vi "AlliGator Compute (1-G2_INT)xMean(INT) Images.vi"(4 "INT Images":T1[](array[typedef]), 6 "Sum(INT)":T1, 7 "G2 Images":T1[](array[typedef]), 8 "Error In":errorcluster, 9 "Min(G2)":T1, 10 "Max(G2)":T1, 11 "Sum(G2)":T1) -> (0 "Error Out":errorcluster, 1 "Min((1-G2/INT)*<INT>)":T1, 2 "Max((1-G2/INT)*<INT>)":T1, 3 "Sum((1-G2/INT)*<INT>)":T1, 5 "(1-G2/INT)*<INT> Images":T1[](array[typedef]))   [LabVIEW 2021, in "AlliGator Dual-Channel Datasets.lvlib"]
doc: "Computes (1 - G2/INT)*<INT>."
uses:
  AlliGator Dual-Channel Datasets.lvlib
  <vilib>/vision/Image Controls.llb/IMAQ Image.ctl
  <vilib>/vision/NI_Vision_Development_Module.lvlib
  Image/Image.lvlib
  Utilities/Utilities.lvlib
panel:
  # "see the AlliGator License on the block diagram (Ctrl+E or Window:Show Block Diagram)"
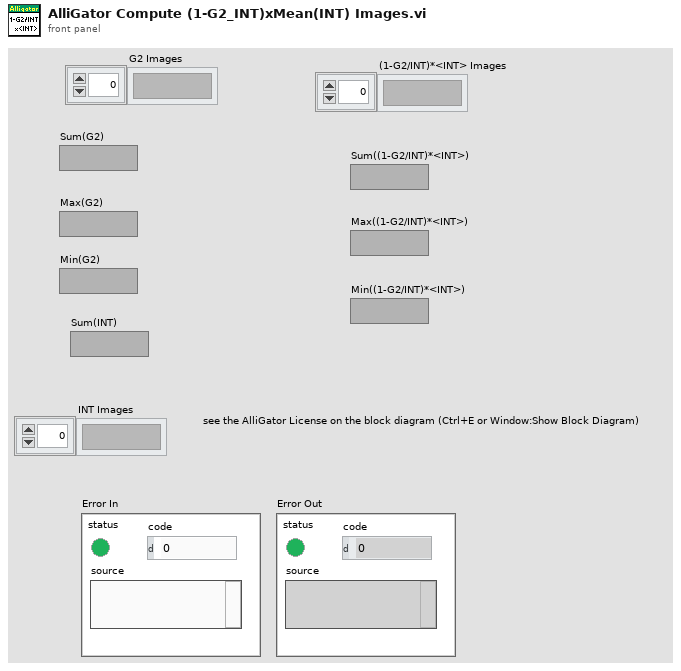
[diagram p1: front panel]
types:
  T1 = typedef "IMAQ Image.ctl" = refnum<image>
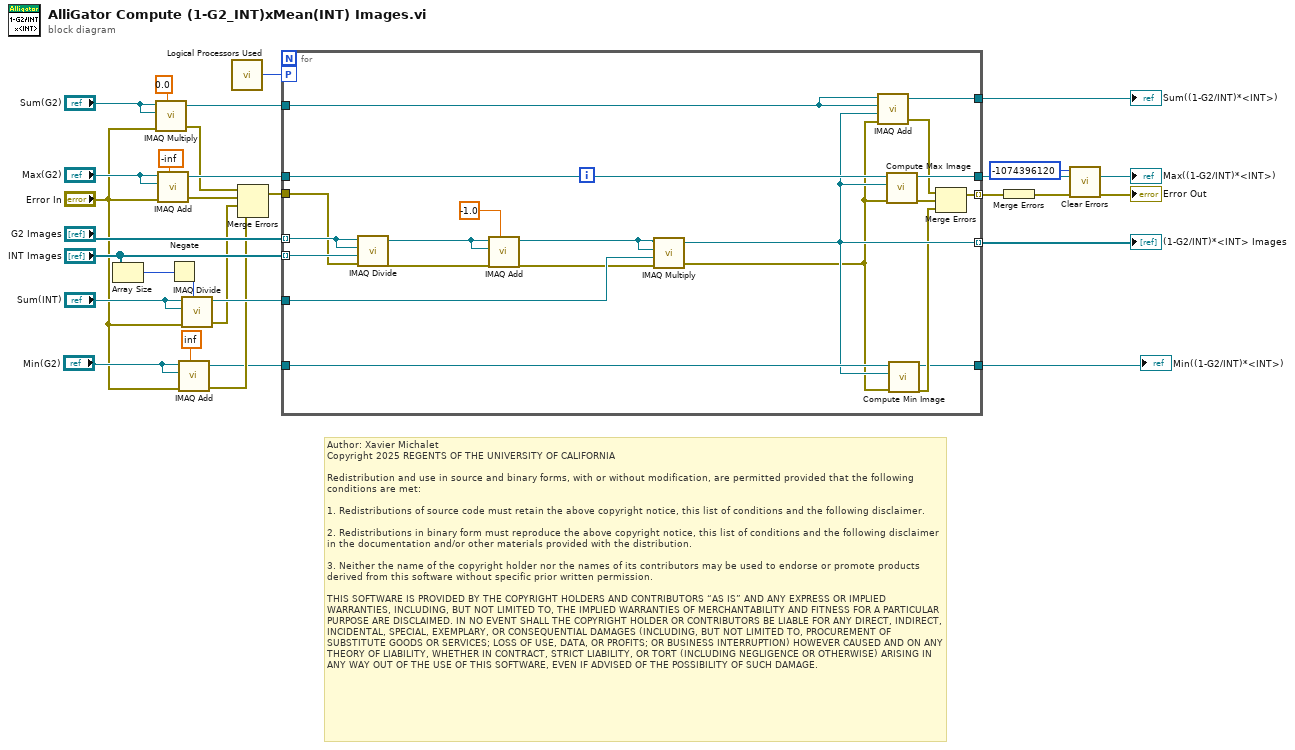
[diagram p0: block diagram]
diagram:
  # "Author: Xavier Michalet\nCopyright 2025 REGENTS OF THE UNIVERSITY OF CALIFORNIA\n\nRedistribution and use in source and binary forms, with or without modification, are permitted provided that the following conditions are met:\n\n1. Redistributions of source code must retain the above copyright notice, this list of conditions and the following disclaimer.\n\n2. Redistributions in binary form must reproduce the above copyright notice, this list of conditions and the following disclaimer in the documentation and/or other materials provided with the distribution.\n\n3. Neither the name of the copyright holder nor the names of its contributors may be used to endorse or promote products derived from this software without specific prior written permission.\n\nTHIS SOFTWARE IS PROVIDED BY THE COPYRIGHT HOLDERS AND CONTRIBUTORS “AS IS” AND ANY EXPRESS OR IMPLIED WARRANTIES, INCLUDING, BUT NOT LIMITED TO, THE IMPLIED WARRANTIES OF MERCHANTABILITY AND FITNESS FOR A PARTICULAR PURPOSE ARE DISCLAIMED. IN NO EVENT SHALL THE COPYRIGHT HOLDER OR CONTRIBUTORS BE LIABLE FOR ANY DIRECT, INDIRECT, INCIDENTAL, SPECIAL, EXEMPLARY, OR CONSEQUENTIAL DAMAGES (INCLUDING, BUT NOT LIMITED TO, PROCUREMENT OF SUBSTITUTE GOODS OR SERVICES; LOSS OF USE, DATA, OR PROFITS; OR BUSINESS INTERRUPTION) HOWEVER CAUSED AND ON ANY THEORY OF LIABILITY, WHETHER IN CONTRACT, STRICT LIABILITY, OR TORT (INCLUDING NEGLIGENCE OR OTHERWISE) ARISING IN ANY WAY OUT OF THE USE OF THIS SOFTWARE, EVEN IF ADVISED OF THE POSSIBILITY OF SUCH DAMAGE."
  n1 = Array Size(array="INT Images") -> (size(s)=w9:i32)
  n2 = call "IMAQ Multiply"("Image Src A"="Sum(G2)", "Constant"=0.0, "Image Dst"="Sum(G2)", "error in (no error)"="Error In") -> ("Image Dst Out"=w26:T1, "error out"=w19:errorcluster)  [unwired: 3 in]
  n3 = call "IMAQ Add"("Image Src A"="Max(G2)", "Constant"=-inf, "Image Dst"="Max(G2)", "error in (no error)"="Error In") -> ("Image Dst Out"=w30:T1, "error out"=w21:errorcluster)  [unwired: 3 in]
  n4 = Negate(x=w9) -> (-x=w11:i32)
  n5 = call "IMAQ Add"("Image Src A"="Min(G2)", "Constant"=inf, "Image Dst"="Min(G2)", "error in (no error)"="Error In") -> ("Image Dst Out"=w2:T1, "error out"=w3:errorcluster)  [unwired: 3 in]
  n6 = call "IMAQ Divide"("Image Src A"="Sum(INT)", "Constant"=w11, "Image Dst"="Sum(INT)", "error in (no error)"="Error In") -> ("Image Dst Out"=w15:T1, "error out"=w12:errorcluster)  [unwired: 3 in]
  n7 = call "Logical Processors Used.vi"() -> ("# Logical Processor Used"=w10:i32)  [unwired: 6 in]
  n8 = Merge Errors(w19, w21, w12, w3) -> (w20:errorcluster)
  n9 = for {
    tunnel: "INT Images" -> [w44] mode=indexing
    tunnel: "G2 Images" -> [w48] mode=indexing
    workers-P: w10 -> [_]
    tunnel: w30 -> [w51]
    tunnel: [w50] -> w22
    tunnel: [w49] -> w18 mode=indexing
    tunnel: w15 -> [w47]
    tunnel: [w34] -> w23 mode=indexing
    tunnel: w26 -> [w46]
    tunnel: [w45] -> w24
    tunnel: w20 -> [w43]
    tunnel: w2 -> [w35]
    tunnel: [w31] -> w1
    n10 = call "IMAQ Divide"("Image Src A"=w48, "Image Dst"=w48, "Image Src B"=w44, "error in (no error)"=w43) -> ("Image Dst Out"=w36:T1, "error out"=w40:errorcluster)  [unwired: 3 in]
    n11 = call "IMAQ Add"("Image Src A"=w36, "Constant"=-1.0, "Image Dst"=w36, "error in (no error)"=w40) -> ("Image Dst Out"=w39:T1, "error out"=w38:errorcluster)  [unwired: 3 in]
    n12 = call "IMAQ Multiply"("Image Src A"=w39, "Image Dst"=w39, "Image Src B"=w47, "error in (no error)"=w38) -> ("Image Dst Out"=w34:T1, "error out"=w33:errorcluster)  [unwired: 3 in]
    n13 = call "IMAQ Add"("Image Src A"=w46, "Image Dst"=w46, "Image Src B"=w34, "error in (no error)"=w33) -> ("Image Dst Out"=w45:T1, "error out"=w41:errorcluster)  [unwired: 3 in]
    n14 = call "Compute Max Image.vi"("error in (no error)"=w33, "New Image"=w34, "Max Image Dst"=w51) -> ("error out"=w42:errorcluster, "Max Image"=w50:T1)  [unwired: 7 in]
    n15 = call "Compute Min Image.vi"("error in (no error)"=w33, "New Image"=w34, "Min Image Dst"=w35) -> ("error out"=w32:errorcluster, "Min Image"=w31:T1)  [unwired: 7 in]
    n16 = Merge Errors(w41, w42, w32) -> (w49:errorcluster)
  }
  "Sum((1-G2/INT)*<INT>)" <- w24
  "(1-G2/INT)*<INT> Images" <- w23
  "Max((1-G2/INT)*<INT>)" <- w22
  "Min((1-G2/INT)*<INT>)" <- w1
  n17 = Merge Errors(w18) -> (w17:errorcluster)
  n18 = call <vilib>:"Clear Errors.vi"("error in (no error)"=w17, "specific error code to clear (0: all)"=-1074396120) -> ("error out"=→"Error Out":errorcluster)  [unwired: 4 in, 1 out]
